vi "温湿度参数配置.vi"() -> ()   [LabVIEW 2016, in "环境动力监测库.lvlib"]
uses:
  <vilib>/Utility/config.llb/NI_LVConfig.lvlib
panel:
  in  "高温告警启用":bool
  in  "湿度下限告警点":dbl
  in  "湿度上限告警点":dbl
  in  "室温下限告警点":dbl
  in  "室温上限告警点":dbl
  in  "模拟量配置":bool
  # "温湿度参数配置"
  # "℃"
  # "℃"
  # "%"
  # "%"
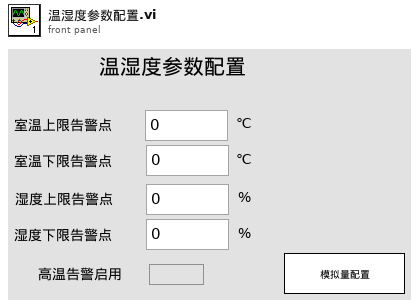
[diagram p1: front panel]
types:
  T1 = typedef "NI_LVConfig.lvlib/Config Data RefNum.ctl" = refnum<k1>
  T2 = cluster{"原始值最小值":dbl, "原始值最大值":dbl, "转换值最小值":dbl, "转换值最大值":dbl, "原始值最小值 2":dbl, "原始值最大值 2":dbl, "转换值最小值 2":dbl, "转换值最大值 2":dbl, "原始值最小值 3":dbl, "原始值最大值 3":dbl, "转换值最小值 3":dbl, "转换值最大值 3":dbl, "原始值最小值 4":dbl, "原始值最大值 4":dbl, "转换值最小值 4":dbl, "转换值最大值 4":dbl, "转换值最大值 5":dbl, "转换值最小值 5":dbl, "原始值最大值 5":dbl, "原始值最小值 5":dbl, "转换值最大值 6":dbl, "转换值最小值 6":dbl, "原始值最大值 6":dbl, "原始值最小值 6":dbl, "转换值最大值 7":dbl, "转换值最小值 7":dbl, "原始值最大值 7":dbl, "原始值最小值 7":dbl, "转换值最大值 8":dbl, "转换值最小值 8":dbl, "原始值最大值 8":dbl, "原始值最小值 8":dbl}
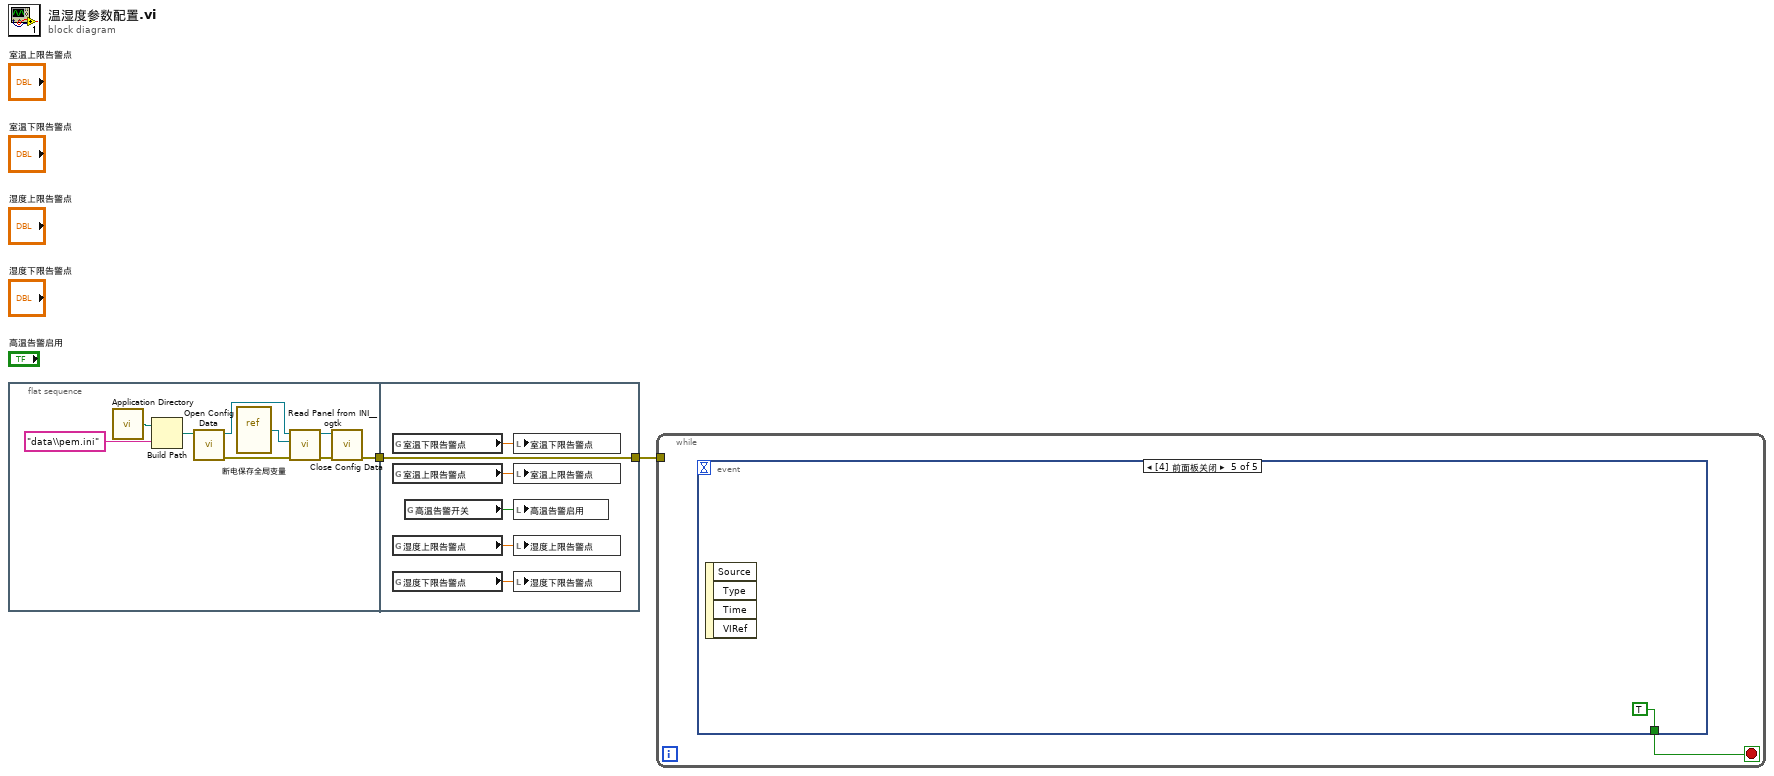
[diagram p0: block diagram]
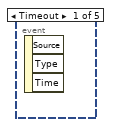
[diagram p2: hidden frame]
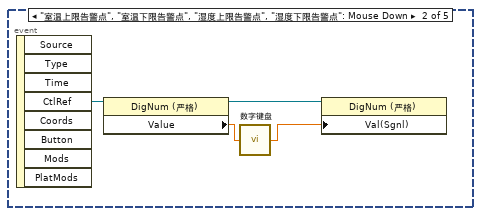
[diagram p3: hidden frame]
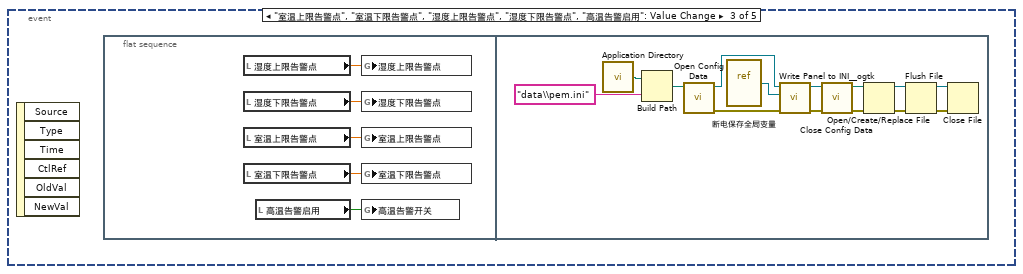
[diagram p4: hidden frame]
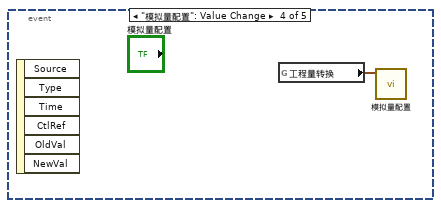
[diagram p5: hidden frame]
diagram:
  n1 = flat-sequence {
    tunnel: [w3] -> w2
    tunnel: [w17] -> w1
    tunnel: w2 -> [w17]
    frame #0 {
      n2 = call <vilib>:"Application Directory.vi"() -> ("Application Directory"=w11:path)
      n3 = Build Path(base path=w11, name or relative path="data\\pem.ini" ("名称或相对路径")) -> (appended path=w9:path)
      n4 = call <vilib>:"Open Config Data.vi"("configuration file path"=w9) -> ("error out"=w5:errorcluster, "refnum"=w8:T1)  [unwired: 8 in, 1 out]
      n5 = vi-ref "断电保存全局变量.vi"() -> (w7:refnum<vi>)
      n6 = call <userlib>:"Read Panel from INI__ogtk.vi"("error in (no error)"=w5, "VI ref"=w7, "refnum"=w8) -> ("error out"=w4:errorcluster, "refnum out"=w6:T1)  [unwired: 7 in]
      n7 = call <vilib>:"Close Config Data.vi"("error in (no error)"=w4, "refnum"=w6) -> ("error out"=w3:errorcluster)  [unwired: 8 in, 1 out]
    }
    frame #1 {
      n8 = global read "断电保存全局变量.vi" "室温下限告警点"() -> (w16:dbl)
      n9 = global read "断电保存全局变量.vi" "室温上限告警点"() -> (w15:dbl)
      n10 = global read "断电保存全局变量.vi" "湿度上限告警点"() -> (w13:dbl)
      n11 = global read "断电保存全局变量.vi" "湿度下限告警点"() -> (w14:dbl)
      n12 = global read "断电保存全局变量.vi" "高温告警开关"() -> (w12:bool)
      n13 = local write "室温下限告警点"(w16) -> ()
      n14 = local write "室温上限告警点"(w15) -> ()
      n15 = local write "高温告警启用"(w12) -> ()
      n16 = local write "湿度上限告警点"(w13) -> ()
      n17 = local write "湿度下限告警点"(w14) -> ()
    }
  }
  n18 = while {
    tunnel: w1 -> [_]
    stop <- w18 stop-if-true
    n19 = event shown="[4] 前面板关闭" {
      selector: _ -> [_ _ _ _ _]
      dyn-events: _ -> [_ _ _ _ _]
      timeout: _ -> [_ _ _ _ _]
      tunnel: [_ _ _ _ TRUE] -> w18
      event Timeout {
        n20 = event-data() -> ()  [unwired: 1 in, 3 out]
      }
      event "室温上限告警点", "室温下限告警点", "湿度上限告警点", "湿度下限告警点": Mouse Down {
        n21 = event-data() -> ("CtlRef"=w19:refnum<vi>)  [unwired: 1 in, 7 out]
        n22 = property class="DigNum (严格)"(reference=w19) -> (reference out=w21:refnum<vi>, "Value"=w22:dbl)  [unwired: 1 in, 1 out]
        n23 = call "数字键盘.vi"("OldNumber"=w22) -> ("NewNumber"=w20:sgl)
        n24 = property class="DigNum (严格)"(reference=w21, "Val(Sgnl)"=w20) -> ()  [unwired: 1 in, 2 out]
      }
      event "室温上限告警点", "室温下限告警点", "湿度上限告警点", "湿度下限告警点", "高温告警启用": Value Change {
        n25 = event-data() -> ()  [unwired: 1 in, 6 out]
        n26 = flat-sequence {
          frame #0 {
            n27 = local read "湿度上限告警点"() -> (w27:dbl)
            n28 = local read "湿度下限告警点"() -> (w26:dbl)
            n29 = local read "室温上限告警点"() -> (w25:dbl)
            n30 = local read "室温下限告警点"() -> (w24:dbl)
            n31 = local read "高温告警启用"() -> (w23:bool)
            n32 = global write "断电保存全局变量.vi" "湿度上限告警点"(w27) -> ()
            n33 = global write "断电保存全局变量.vi" "湿度下限告警点"(w26) -> ()
            n34 = global write "断电保存全局变量.vi" "室温上限告警点"(w25) -> ()
            n35 = global write "断电保存全局变量.vi" "室温下限告警点"(w24) -> ()
            n36 = global write "断电保存全局变量.vi" "高温告警开关"(w23) -> ()
          }
          frame #1 {
            n37 = call <vilib>:"Application Directory.vi"() -> ("Application Directory"=w40:path)
            n38 = Build Path(base path=w40, name or relative path="data\\pem.ini" ("名称或相对路径")) -> (appended path=w39:path)
            n39 = call <vilib>:"Open Config Data.vi"("configuration file path"=w39) -> ("error out"=w35:errorcluster, "refnum"=w38:T1)  [unwired: 8 in, 1 out]
            n40 = vi-ref "断电保存全局变量.vi"() -> (w37:refnum<vi>)
            n41 = call <userlib>:"Write Panel to INI__ogtk.vi"("error in (no error)"=w35, "VI ref"=w37, "refnum"=w38) -> ("error out"=w34:errorcluster, "refnum out"=w36:T1)  [unwired: 7 in]
            n42 = call <vilib>:"Close Config Data.vi"("error in (no error)"=w34, "refnum"=w36) -> ("error out"=w29:errorcluster, "file path"=w28:path)  [unwired: 8 in]
            n43 = Open/Create/Replace File(file path (use dialog)=w28, error in=w29) -> (refnum out=w32:refnum<file>, error out=w33:errorcluster)  [unwired: 4 in, 1 out]
            n44 = Flush File(refnum=w32, error in=w33) -> (refnum out=w31:refnum<file>, error out=w30:errorcluster)
            n45 = Close File(refnum=w31, error in=w30) -> ()  [unwired: 2 out]
          }
        }
      }
      event "模拟量配置": Value Change {
        n46 = event-data() -> ()  [unwired: 1 in, 6 out]
        n47 = global read "通讯全局变量断电保存.vi" "工程量转换"() -> (w42:T2)
        n48 = call "模拟量配置.vi"("工程量转换"=w42) -> ()  [unwired: 11 in]
      }
      event Panel Close {
        n49 = event-data() -> ()  [unwired: 1 in, 4 out]
      }
    }
  }
